vi "Generate Counter Updated Event.vi"(8 "error in (no error)":errorcluster, 10 "Count":dbl, 11 "Counter in":refnum<class "Counter.lvclass">) -> (0 "error out":errorcluster)   [LabVIEW 2018, in "Counter.lvlib" / "Counter.lvclass"]
uses:
  Counter.lvclass
  Counter.lvclass/Counter.ctl
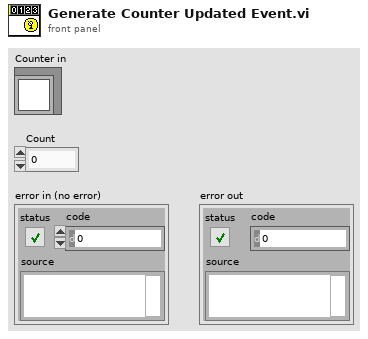
[diagram p1: front panel]
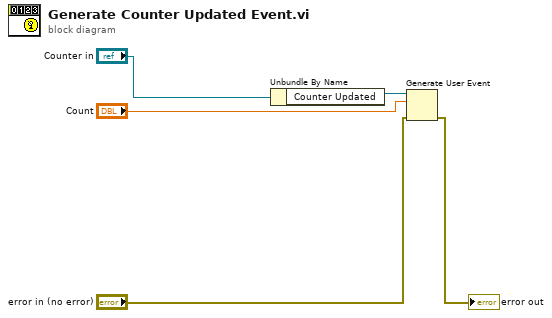
[diagram p0: block diagram]
diagram:
  n1 = Unbundle By Name("Counter in") -> ("Counter Updated"=w2:refnum<user-event>)
  n2 = Generate User Event(user event=w2, event data cluster="Count", error in="error in (no error)") -> (error out=→"error out":errorcluster)  [unwired: 1 in, 1 out]
